vi "Get Paths.vi"(11 "Path IN":path) -> (3 "App Path":path)   [LabVIEW 2023]
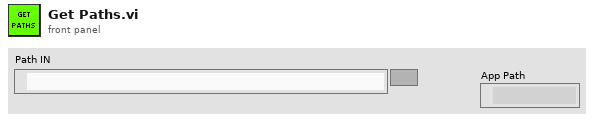
[diagram p1: front panel]
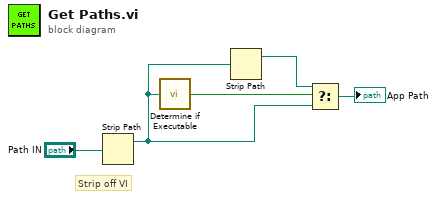
[diagram p0: block diagram]
diagram:
  # "Strip off VI"
  n1 = Strip Path(path="Path IN") -> (stripped path=w1:path)  [unwired: 1 out]
  n2 = call "Determine if Executable.vi"("Path"=w1) -> ("EXE?"=w5:bool)
  n3 = Strip Path(path=w1) -> (stripped path=w3:path)  [unwired: 1 out]
  n4 = Select(t=w3, s=w5, f=w1) -> (s? t:f=→"App Path":path)
